vi "Switch Configure.vi"(7 "Resistivity":T1, 8 "error in (no error)":errorcluster, 11 "VISA resource name in":refnum<visa-resource-name>) -> (0 "error out":errorcluster, 3 "VISA resource name out":refnum<visa-resource-name>)   [LabVIEW 2016, in "Hall Effect Library.lvlib"]
uses:
  Hall Effect Library.lvlib
  Public/Controls/Resisitivity.ctl
  Global Variables/Instruments.vi
  Switch Configure (3706).vi
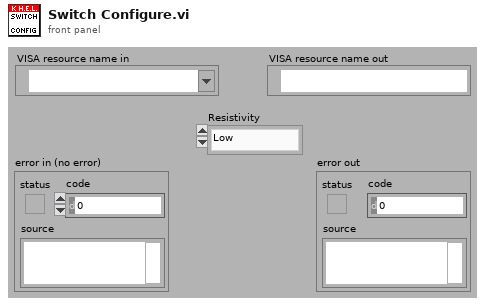
[diagram p1: front panel]
types:
  T1 = typedef "Hall Effect Library.lvlib/Resisitivity.ctl" = enum16{"Low", "High"}
  T2 = typedef "Hall Effect Library.lvlib/Switches.ctl" = enum16{"3706A"}
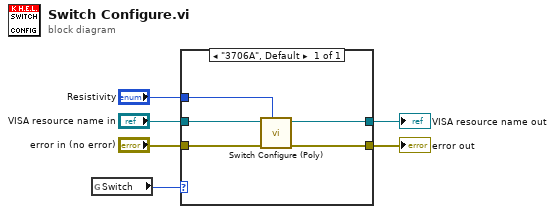
[diagram p0: block diagram]
diagram:
  n1 = global read "Instruments.vi" "Switch"() -> (w6:T2)
  n2 = case shown="\"3706A\", Default" w6 {
    tunnel: "VISA resource name in" -> [w11]
    tunnel: "error in (no error)" -> [w10]
    tunnel: [w9] -> w2
    tunnel: [w8] -> w1
    tunnel: "Resistivity" -> [w7]
    frame "3706A", Default {
      n3 = call-poly "Switch Configure (Poly).vi"("Resistivity"=w7, "error in (no error)"=w10, "VISA resource name in"=w11) -> ("error out"=w9:errorcluster, "VISA resource name out"=w8:refnum<visa-resource-name>)  [unwired: 7 out]
    }
  }
  "error out" <- w2
  "VISA resource name out" <- w1
